vi "New Client Handle.vi"(4 "headers":T1[](array[typedef]), 6 "verify server(true)":bool=TRUE, 7 "cookie file":path, 8 "error in (no error)":errorcluster, 9 "password":string, 10 "username":string, 11 "REST Client in":refnum<class "REST Client_JKI.lvclass">) -> (0 "error out":errorcluster, 2 "client handle out":T2, 3 "REST Client out":refnum<class "REST Client_JKI.lvclass">)   [LabVIEW 2018, in "REST Client_JKI.lvlib" / "REST Client_JKI.lvclass"]
uses:
  REST Client_JKI.lvclass
  <vilib>/httpClient/ClientHandle.ctl
  REST Client/HTTP Header.ctl
  <vilib>/httpClient/LabVIEWHTTPClient.lvlib
  REST Client/REST Client.lvclass
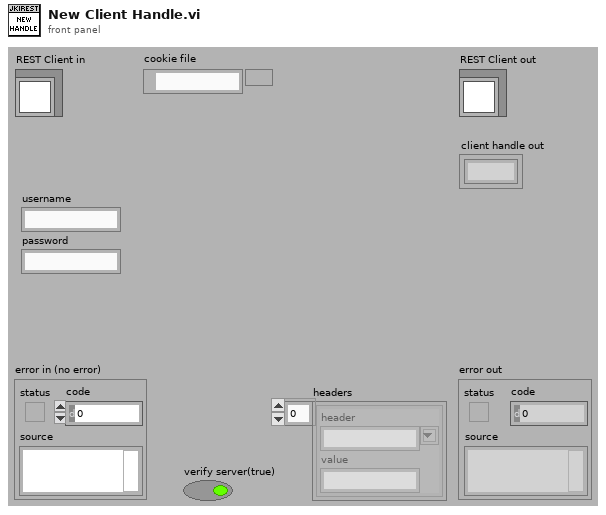
[diagram p1: front panel]
types:
  T1 = typedef "REST Client_JKI.lvlib/REST Client.lvclass/HTTP Header.ctl" = cluster{"header":string, "value":string}
  T2 = typedef "LabVIEWHTTPClient.lvlib/ClientHandle.ctl" = refnum<k1>
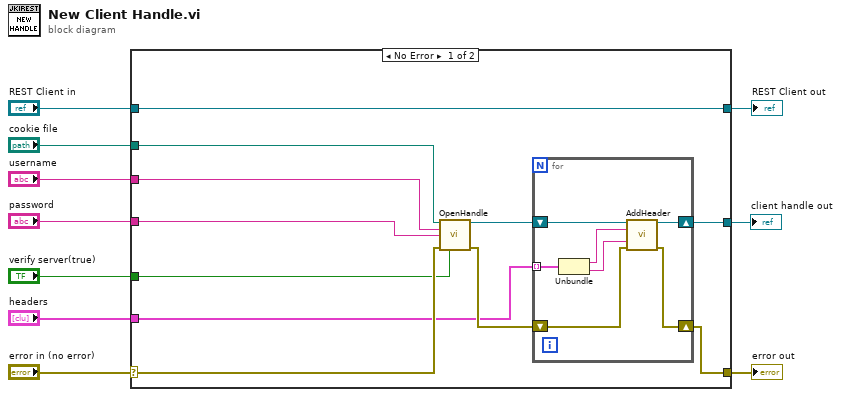
[diagram p0: block diagram]
diagram:
  n1 = case shown="No Error" "error in (no error)" {
    selector: "error in (no error)" -> [w20 w30]
    tunnel: [w13 w30] -> w9
    tunnel: [w21 w29] -> w7
    tunnel: "REST Client in" -> [w21 w29]
    tunnel: "cookie file" -> [w19 _]
    tunnel: "username" -> [w18 _]
    tunnel: "password" -> [w17 _]
    tunnel: "verify server(true)" -> [w16 _]
    tunnel: [w14 _] -> w2
    tunnel: "headers" -> [w11 _]
    frame No Error {
      n2 = call <vilib>:"OpenHandle.vi"("cookie file"=w19, "username"=w18, "password"=w17, "error in (no error)"=w20, "verify server(true)"=w16) -> ("client handle out"=w15:T2, "error out"=w12:errorcluster)  [unwired: 9 in]
      n3 = for {
        shift-right: [w26] -> w13
        shift-left: w12 -> [w25]
        shift-right: [w27] -> w14
        shift-left: w15 -> [w28]
        tunnel: w11 -> [w24] mode=indexing
        n4 = Unbundle(w24) -> ("header"=w23:string, "value"=w22:string)
        n5 = call <vilib>:"AddHeader.vi"("client handle"=w28, "header"=w23, "value"=w22, "error in (no error)"=w25) -> ("client handle out"=w27:T2, "error out"=w26:errorcluster)  [unwired: 10 in]
      }
    }
    frame Error {
    }
  }
  "error out" <- w9
  "REST Client out" <- w7
  "client handle out" <- w2
